vi "Fowlkes_Mallows_Score.vi"(8 "error in (no error)":errorcluster caption="entrée d'erreur (pas d'erreur)", 9 "labels_pred":string[][](array[string]), 10 "labels_true":string[][](array[string]), 11 "fowlkes_mallows_score":cluster{"sparse":bool}) -> (0 "error out":errorcluster caption="sortie d'erreur", 3 "String Data":string)   [LabVIEW 2020]
doc: "Measure the similarity of two clusterings of a set of points.\n\n\nThe Fowlkes-Mallows index (FMI) is defined as the geometric mean between of the precision and recall :\n\nFMI = TP / sqrt((TP + FP) * (TP + FN))\n\nWhere TP is the number of True Positive (i.e. the number of pair of points that belongs in the same clusters in both labels_true and labels_pred), FP is the number of False Positive (i.e. the number of pair of points that belongs in the same clusters in labels_true and not in labels_pred) and FN is the number of False Negative (i.e the number of pair of points that belongs in the same clusters in labels_pred and not in labels_True).\n\nThe score ranges from 0 to 1. A high value indicates a good similarity between two clusters.\n\n\n\nParameters :\n\n- labels_true : int array, shape = (n_samples,)\nA clustering of the data into disjoint subsets.\n\n- labels_pred : array, shape = (n_samples, )\nA clustering of the data into disjoint subsets.\n\n- sparse : bool\nCompute contingency matrix internally with sparse matrix.\n\nReturns :\n\n- score : float\nThe resulting Fowlkes-Mallows score."
uses:
  Fowlkes_Mallows_Score.lvclass
panel:
  out "Fowlkes_Mallows_Score.lvclass":refnum<class "Fowlkes_Mallows_Score.lvclass">
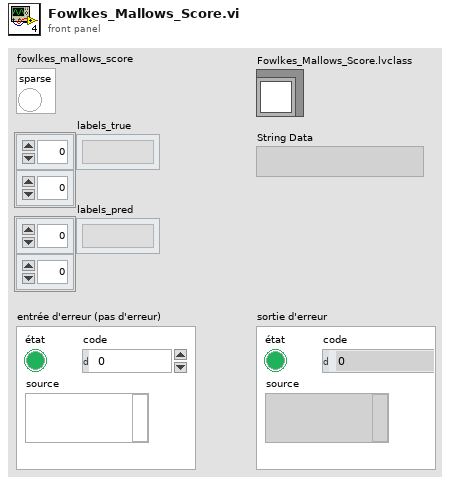
[diagram p1: front panel]
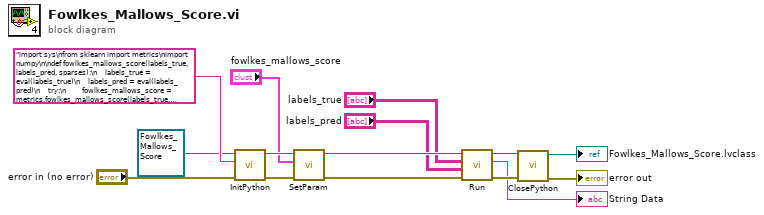
[diagram p0: block diagram]
diagram:
  n1 = call-dynamic "InitPython.vi"("error in (no error)"="error in (no error)", "Python Instruction"="import sys\nfrom sklearn import metrics\nimport numpy\n\ndef fowlkes_mallows_score(labels_true, labels_pred, sparses):\n    labels_true = eval(labels_true)\n    labels_pred = eval(labels_pred)\n    try:\n        fowlkes_mallows_score = metrics.fowlkes_mallows_score(labels_true, labels_pred, sparses)\n        fowlkes_mallows_score = fowlkes_mallows_score.tolist()\n        return str(fowlkes_mallows_score)\n    except:\n        erreur = sys.exc_info()\n        typerr = u\"%s\" % (erreur[0])\n        typerr = typerr[typerr.find(\"'\")+1:typerr.rfind(\"'\")]\n        msgerr = u\"%s\" % (erreur[1])\n        message = str('/!\\\\ {0} : {1}'. format(typerr,msgerr))\n        return message", "Scikit-learn en entrée"=refnum<class "Fowlkes_Mallows_Score.lvclass"> refnum ("Fowlkes_Mallows_Score.lvclass")) -> ("error out"=w11:errorcluster, "Scikit-learn en sortie"=w12:refnum<class "Fowlkes_Mallows_Score.lvclass">)  [unwired: 7 in]
  n2 = call-dynamic "SetParam.vi"("error in (no error)"=w11, "fowlkes_mallows_score"="fowlkes_mallows_score", "Fowlkes_Mallows_Score.lvclass"=w12) -> ("error out"=w7:errorcluster, "Fowlkes_Mallows_Score.lvclass"=w8:refnum<class "Fowlkes_Mallows_Score.lvclass">)  [unwired: 7 in]
  n3 = call-dynamic "Run.vi"("error in (no error)"=w7, "labels_pred"="labels_pred", "labels_true"="labels_true", "Fowlkes_Mallows_Score.lvclass"=w8) -> ("error out"=w5:errorcluster, "String Data"=→"String Data":string, "Fowlkes_Mallows_Score.lvclass"=w6:refnum<class "Fowlkes_Mallows_Score.lvclass">)  [unwired: 5 in]
  n4 = call-dynamic "ClosePython.vi"("error in (no error)"=w5, "Scikit-learn en entrée"=w6) -> ("error out"=→"error out":errorcluster, "Scikit-learn en sortie"=→"Fowlkes_Mallows_Score.lvclass":refnum<class "Fowlkes_Mallows_Score.lvclass">)  [unwired: 8 in]
